vi "Grid_Main_dev.vi"(9 "DC images in":dbl[][][](array[numeric]), 10 "Part of multigrid":bool, 11 "Settings":T3={"Drift Correction Settings"={"Drift Correction every"=80, "Drift correction Pixels"=256, "Channel index (0-23)"=0, "MaxImagesBack"=2, "Threshold"=2, "Increment"=8, "max applied Drift Correction"=20, "Correct Drift"=TRUE, "Correlate"=0, "Correct z drift"=FALSE, "zdrift \nDuration (s)"=0.0}, "Spectroscopy Setting"={"Imaging Current"=1e-11, "ref Current"=7e-11, "tip Speed (m/s)"=2e-09, "Imaging Bias"=0.02, "ref Bias"=-0.1, "preSTS delay [ms]"=500, "STS z offset"=2e-10, "during Spec Bias (V)"=-0.1, "trigger1 < Hz"=0.0, "trigger 2 >Hz"=0.0, "autoStop"=FALSE, "Spectroscopy"=0, "PLL ON/OFF"=TRUE, "readjust setpoint every "=1, "z Reference (constHeight)"=FALSE, "Lock In"=TRUE}, "Misc"={"File name"="symmetric_node_zOff=200p", "Email when finished"="cornelius.krull@monash.edu,Dhaneesh.Gopalakrishnan@monash.edu,marina.castelli@monash.edu"}, "Grid Settings"={"type"=1, "type order"=1, "X pixel"=0, "Y pixel"=0, "Grid_Parms"={"center X (m)"=0.0, "center Y (m)"=0.0, "width (m)"=0.0, "height (m)"=0.0, "angle (deg)"=0.0}}} {"Grid Settings"."type order" items=["Grid", "Random", "Adam7"]; "Grid Settings"."type" items=["Line", "Grid", "Cloud"]; "Spectroscopy Setting"."Spectroscopy" items=["Bias", "zSpec"]; "Spectroscopy Setting"."trigger 2 >Hz" format="%#_6p"; "Spectroscopy Setting"."trigger1 < Hz" format="%#_6p"; "Spectroscopy Setting"."during Spec Bias (V)" format="%#_5p"; "Spectroscopy Setting"."STS z offset" format="%#_6p"; "Spectroscopy Setting"."ref Bias" format="%#_6p"; "Spectroscopy Setting"."Imaging Bias" format="%#_6p"; "Spectroscopy Setting"."tip Speed (m/s)" format="%.2p"; "Spectroscopy Setting"."ref Current" format="%#_6p"; "Spectroscopy Setting"."Imaging Current" format="%#_6p"; "Drift Correction Settings"."Correlate" items=["first Frame", "successive Frames"]; "Drift Correction Settings"."max applied Drift Correction" min=1 max=100 step=1 format="%.0p"; "Drift Correction Settings"."Threshold" min=1 step=1; "Drift Correction Settings"."Channel index (0-23)" items=["Current"=0, "Z (m)"=14]}) -> (1 "DC images out":dbl[][][](array[numeric]), 3 "Settings out":T2)   [LabVIEW 2014]
uses:
  <userlib>/Nanonis Prog Interface V5/Nanonis Prog Interface.lvlib
panel:
  in  "topo_pixel":i32
  in  "resume":T1
  in  "stop":bool
  out "total points":i32
  out "Points taken":i32
  out "ETA":timestamp=timestamp(3575267058.899443 s since 1904-01-01)
  out "remaining time":dbl format="%<%H:%M:%S>t"
  out "Progress":u8(slide)=100 scale=0.0..100.0 scale format="%#.1g"
  out "Last z adjustment":dbl
  out "Last Drift detected (images back)":i32
  out "Y Offset out":sgl format="%#_6p"
  out "X Offset out":sgl format="%#_6p"
  out "Drift Correction Image":picture
  # "RUN smart tilt before starting the GRID\nCHECK CUTOFF\nmove tip to reference point for tip height"
  # "%"
  # "finish the last action and then"
  # "GRID points"
  # "Increase this if no Drift was detected for \na certain number of images"
  # "% of image size"
  # "Only first frame works"
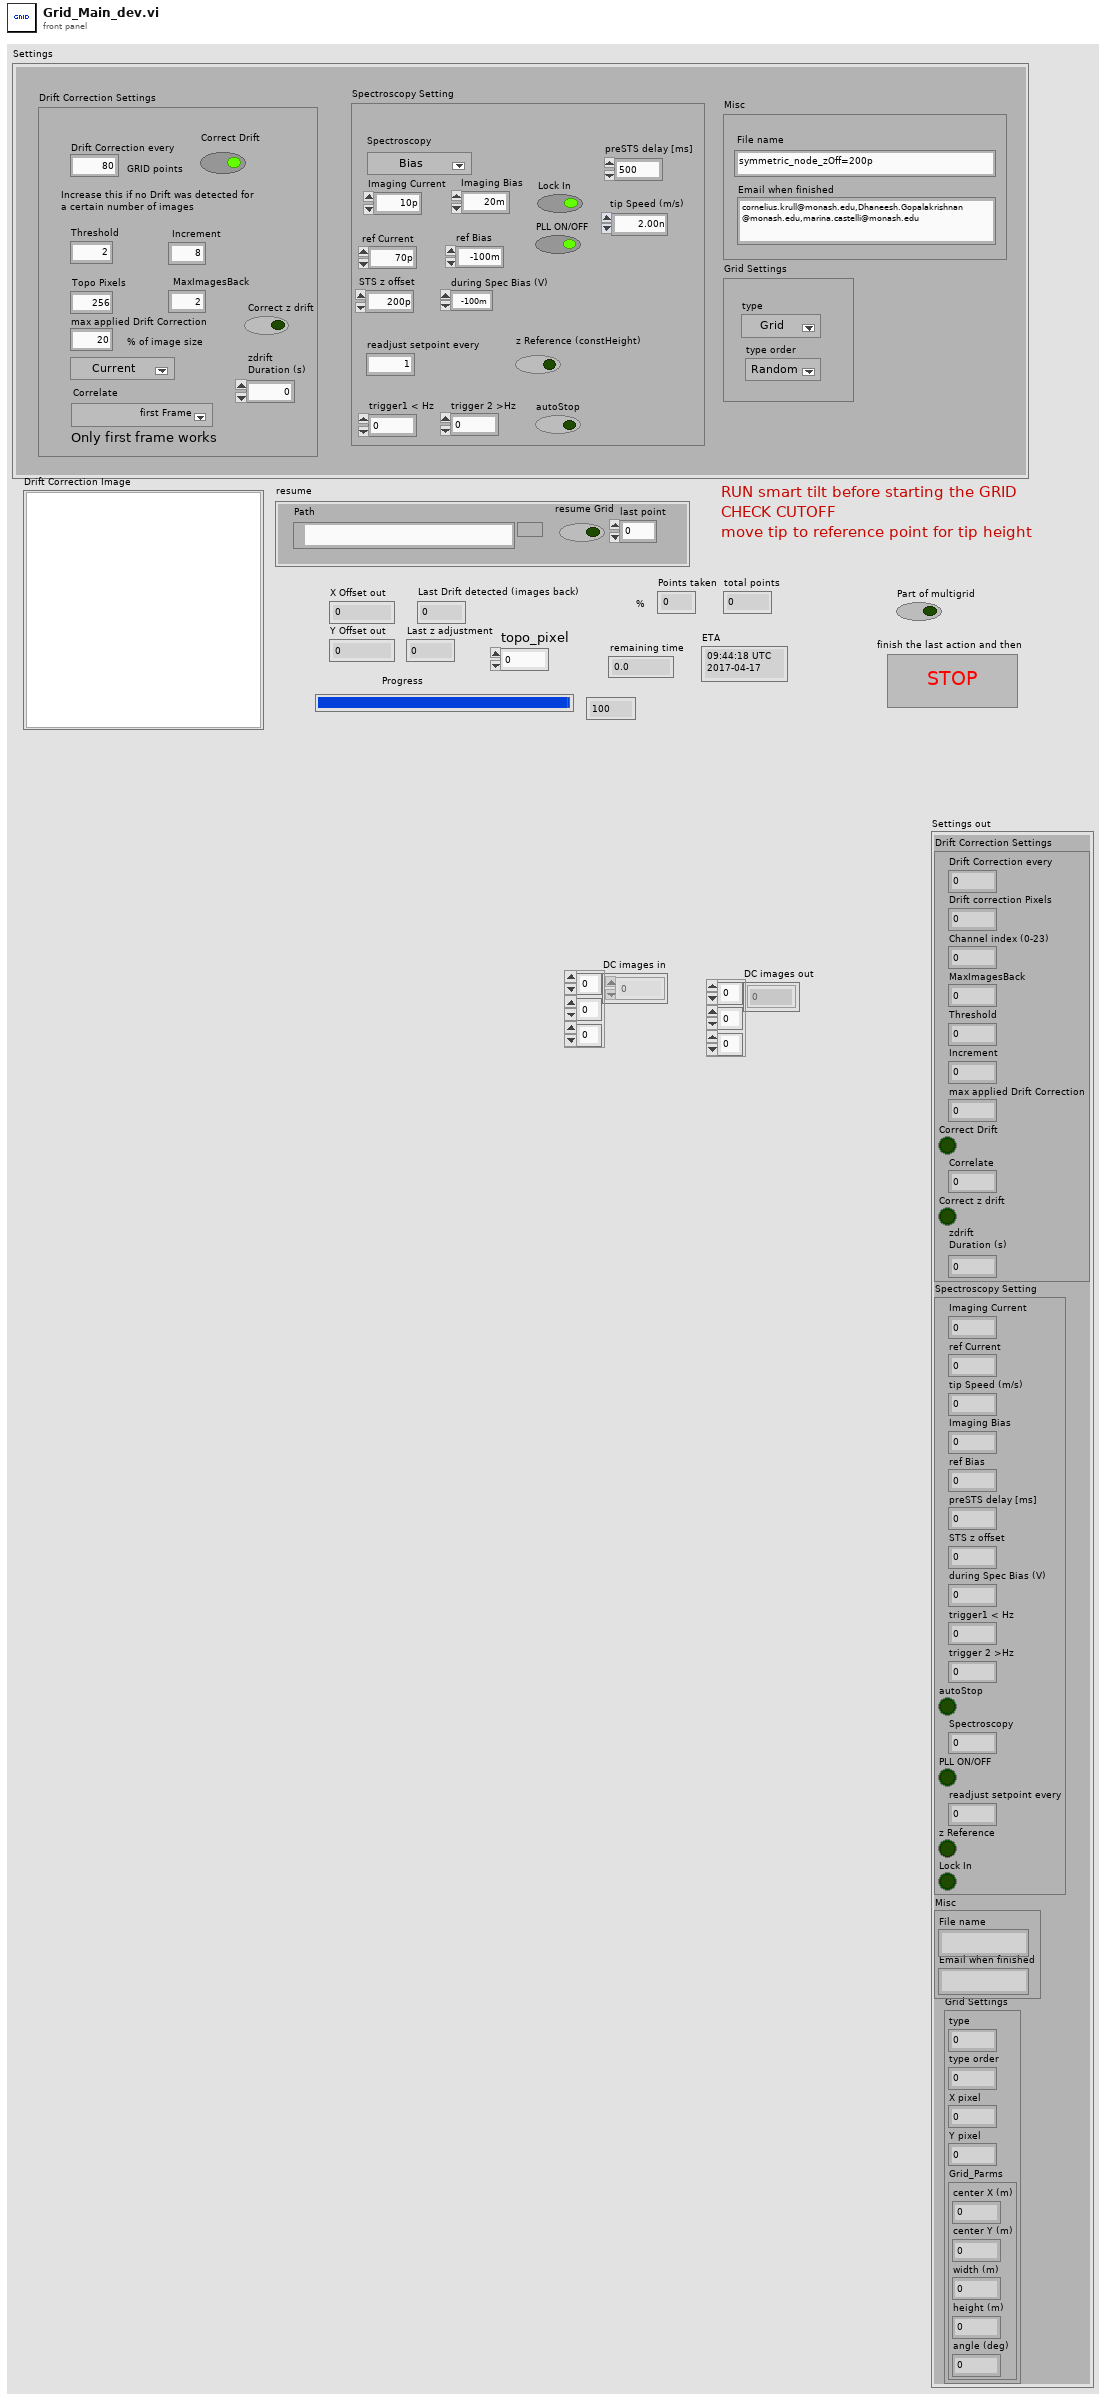
[diagram p1: front panel]
types:
  T1 = cluster{"resume Grid":bool, "Path":path, "last point":i32}
  T2 = cluster{"Drift Correction Settings":cluster{"Drift Correction every":i32, "Drift correction Pixels":i32, "Channel index (0-23)":u8, "MaxImagesBack":i32, "Threshold":i32, "Increment":i32, "max applied Drift Correction":i32, "Correct Drift":bool, "Correlate":u16, "Correct z drift":bool, "zdrift \nDuration (s)":dbl}, "Spectroscopy Setting":cluster{"Imaging Current":dbl, "ref Current":dbl, "tip Speed (m/s)":sgl, "Imaging Bias":dbl, "ref Bias":dbl, "preSTS delay [ms]":u32, "STS z offset":dbl, "during Spec Bias (V)":sgl, "trigger1 < Hz":sgl, "trigger 2 >Hz":sgl, "autoStop":bool, "Spectroscopy":u16, "PLL ON/OFF":bool, "readjust setpoint every ":i32, "z Reference":bool, "Lock In":bool}, "Misc":cluster{"File name":string, "Email when finished":string}, "Grid Settings":cluster{"type":u16, "type order":u16, "X pixel":i32, "Y pixel":i32, "Grid_Parms":cluster{"center X (m)":sgl, "center Y (m)":sgl, "width (m)":sgl, "height (m)":sgl, "angle (deg)":sgl}}}
  T3 = cluster{"Drift Correction Settings":cluster{"Drift Correction every":i32, "Drift correction Pixels":i32, "Channel index (0-23)":u8, "MaxImagesBack":i32, "Threshold":i32, "Increment":i32, "max applied Drift Correction":i32, "Correct Drift":bool, "Correlate":u16, "Correct z drift":bool, "zdrift \nDuration (s)":dbl}, "Spectroscopy Setting":cluster{"Imaging Current":dbl, "ref Current":dbl, "tip Speed (m/s)":sgl, "Imaging Bias":dbl, "ref Bias":dbl, "preSTS delay [ms]":u32, "STS z offset":dbl, "during Spec Bias (V)":sgl, "trigger1 < Hz":sgl, "trigger 2 >Hz":sgl, "autoStop":bool, "Spectroscopy":u16, "PLL ON/OFF":bool, "readjust setpoint every ":i32, "z Reference (constHeight)":bool, "Lock In":bool}, "Misc":cluster{"File name":string, "Email when finished":string}, "Grid Settings":cluster{"type":u16, "type order":u16, "X pixel":i32, "Y pixel":i32, "Grid_Parms":cluster{"center X (m)":sgl, "center Y (m)":sgl, "width (m)":sgl, "height (m)":sgl, "angle (deg)":sgl}}}
  T4 = cluster{"Drift File out":refnum<file>, "zFile":refnum<file>, "BinFile ref":refnum<file>, "xyFile":refnum<file>}
  T5 = cluster{"Drift Correction every":i32, "Drift correction Pixels":i32, "Channel index (0-23)":u8, "MaxImagesBack":i32, "Threshold":i32, "Increment":i32, "max applied Drift Correction":i32, "Correct Drift":bool, "Correlate":u16, "Correct z drift":bool, "zdrift \nDuration (s)":dbl}
  T6 = cluster{"Imaging Current":dbl, "ref Current":dbl, "tip Speed (m/s)":sgl, "Imaging Bias":dbl, "ref Bias":dbl, "preSTS delay [ms]":u32, "STS z offset":dbl, "during Spec Bias (V)":sgl, "trigger1 < Hz":sgl, "trigger 2 >Hz":sgl, "autoStop":bool, "Spectroscopy":u16, "PLL ON/OFF":bool, "readjust setpoint every ":i32, "z Reference":bool, "Lock In":bool}
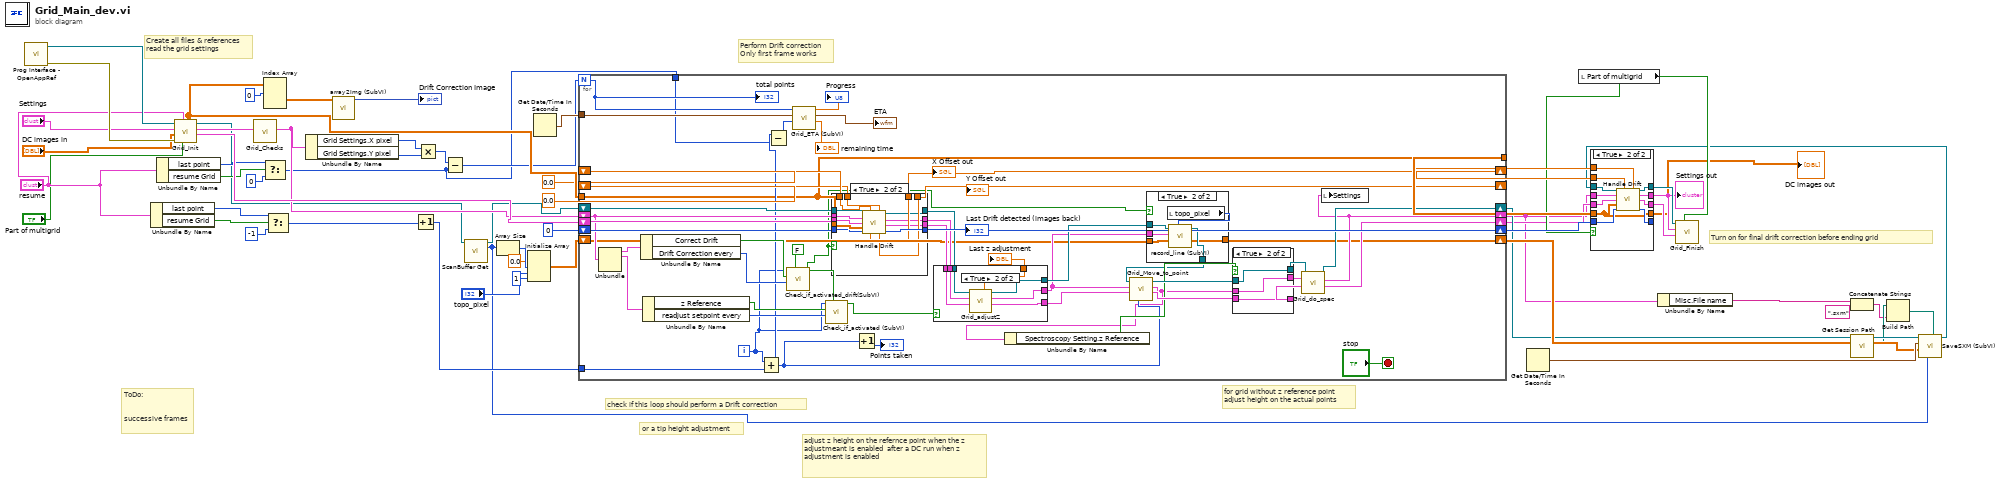
[diagram p0: block diagram]
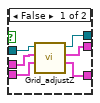
[diagram p4: hidden frame]
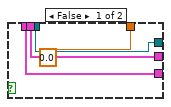
[diagram p5: hidden frame]
diagram:
  # "Turn on for final drift correction before ending grid"
  # "ToDo:\n\n\nsuccessive frames"
  # "Perform Drift correction\nOnly first frame works"
  # "check if this loop should perform a Drift correction"
  # "for grid without z reference point \nadjust height on the actual points"
  # "or a tip height adjustment"
  # "Create all files & references\nread the grid settings"
  # "adjust z height on the refernce point when the z adjustmeant is enabled  after a DC run when z adjustment is enabled"
  n1 = call <userlib>:"Prog Interface - OpenAppRef.vi"() -> ("Error out"=w58:errorcluster, "Application reference"=w59:refnum<vi>)  [unwired: 6 in]
  n2 = Unbundle By Name("resume") -> ("last point"=w41:i32, "resume Grid"=w43:bool)
  n3 = Unbundle By Name("resume") -> ("last point"=w35:i32, "resume Grid"=w37:bool)
  n4 = call "Grid_Init.vi"("Part of multigrid"="Part of multigrid", "resume"="resume", "Error in"=w58, "DC images in"="DC images in", "Settings"="Settings", "Application reference"=w59) -> ("FileRefs"=w56:T4, "Settings out"=w46:T2, "Application ref out"=w18:refnum<vi>, "DC images out"=w54:dbl[][][])  [unwired: 1 in, 1 out]
  n5 = call "Grid_Checks.vi"("Settings"=w46) -> ("Settings out"=w45:T2)  [unwired: 10 in]
  n6 = Index Array(array=w54, index (dim 0)=0 ("index (page)")) -> (element=w55:dbl[][])  [unwired: 2 in]
  n7 = Select(t=w35, s=w37, f=0) -> (s? t:f=w32:i32)
  n8 = Select(t=w41, s=w43, f=-1) -> (s? t:f=w40:i32)
  n9 = Unbundle By Name(w45) -> ("Grid Settings.X pixel"=w49:i32, "Grid Settings.Y pixel"=w48:i32)
  n10 = call "array2Img (SubVI).vi"("Rxy"=w55) -> ("new picture"=→"Drift Correction Image":picture)  [unwired: 10 in]
  n11 = Increment(x=w40) -> (x+1=w38:i32)
  n12 = Multiply(x=w49, y=w48) -> (x*y=w33:i32)
  n13 = Subtract(x=w33, y=w32) -> (x-y=w39:i32)
  n14 = call <userlib>:"ScanBuffer Get.vi"("Application ref in"=w18) -> ("Application ref out"=w17:refnum<vi>, "Channels indexes (0-23)"=w11:i32[])  [unwired: 10 in, 3 out]
  n15 = Array Size(array=w11) -> (size(s)=w20:i32)
  n16 = Initialize Array(0.0 ("element"), w20, "topo_pixel", 1 ("dimension size")) -> (w14:dbl[][][])
  n17 = Get Date/Time In Seconds() -> (seconds since 1Jan1904=w47:timestamp)
  n18 = for {
    N: w39 -> [w73]
    tunnel: w54 -> [w67]
    shift-right: [w108] -> w30
    shift-left: 0 ("Last Drift out") -> [w107]
    shift-right: [w103] -> w28
    shift-left: sgl 0.0 ("X Offset out") -> [w106]
    shift-right: [w104] -> w27
    shift-left: sgl 0.0 ("Y Offset out") -> [w105]
    tunnel: w47 -> [w95]
    shift-right: [w93] -> w9
    shift-left: w17 -> [w109]
    shift-right: [w69] -> w4
    shift-left: w45 -> [w80]
    shift-right: [w92] -> w5
    shift-left: w56 -> [w110]
    tunnel: w38 -> [w81]
    tunnel: w32 -> [w70]
    tunnel: [w67] -> w29
    shift-right: [w62] -> w12
    shift-left: w14 -> [w61]
    i -> [w66]
    stop <- "stop" stop-if-true
    n19 = Unbundle(w80) -> ("Drift Correction Settings"=w79:T5, "Spectroscopy Setting"=w77:T6)  [unwired: 2 out]
    n20 = Unbundle By Name(w79) -> ("Correct Drift"=w78:bool, "Drift Correction every"=w74:i32)
    n21 = Unbundle By Name(w77) -> ("z Reference"=w76:bool, "readjust setpoint every"=w75:i32)
    n22 = Add(x=w66, y=w81) -> (x+y=w71:i32)
    n23 = Subtract(x=w71, y=w70) -> (x-y=w72:i32)
    n24 = call "Check_if_activated_drift(SubVI).vi"("Override"=FALSE, "activate  every  iterations"=w74, "activated?"=w78, "Iteration"=w66) -> ("perform action"=w60:bool)  [unwired: 7 in]
    n25 = call "Grid_ETA (SubVI).vi"("points taken"=w72, "seconds since 1Jan1904"=w95, "points todo"=w73) -> ("Numeric 4"=→"remaining time":dbl, "Time Stamp"=→"ETA":timestamp, "Numeric 3"=→"Progress":dbl)  [unwired: 6 in]
    n26 = call "Check_if_activated (SubVI).vi"("Override"=w60, "activate  every  iterations"=w75, "activated?"=w76, "Iteration"=w66) -> ("perform action"=w100:bool)  [unwired: 7 in]
    n27 = case shown="True" w60 {
      tunnel: w80 -> [w141 w157]
      tunnel: w110 -> [w140 w156]
      tunnel: w109 -> [w139 w155]
      tunnel: w67 -> [_ w154]
      tunnel: [w142 w153] -> w108
      tunnel: w107 -> [w142 w152]
      tunnel: w106 -> [w144 w151]
      tunnel: w105 -> [w143 w150]
      tunnel: [w143 w149] -> w104
      tunnel: [w144 w148] -> w103
      tunnel: [w139 w145] -> w102
      tunnel: [w141 w147] -> w83
      tunnel: [w140 w146] -> w101
      frame False {
      }
      frame True {
        n28 = call "Handle Drift.vi"("Application ref in"=w155, "X Offset in"=w151, "Y Offset In"=w150, "Settings"=w157, "FileRefs"=w156, "Drift Correction image"=w154, "Last Drift"=w152) -> ("Application out"=w145:refnum<vi>, "Settings out"=w147:T2, "FileRefs out File Refs  Out"=w146:T4, "X Offset out"=w148:sgl, "Y Offset out"=w149:sgl, "Last Drift out"=w153:i32)  [unwired: 3 in]
      }
    }
    "X Offset out" <- w103
    "Y Offset out" <- w104
    "Last Drift detected (images back)" <- w108
    n29 = Increment(x=w71) -> (x+1=→"Points taken":i32)
    n30 = case shown="True" w100 {
      tunnel: w102 -> [w130 w138]
      tunnel: w101 -> [w129 w137]
      tunnel: w83 -> [w128 w132]
      tunnel: [w129 w136] -> w94
      tunnel: [w128 w135] -> w63
      tunnel: [w130 w134] -> w65
      tunnel: [0.0 ("Last z adjustment") w133] -> w91
      frame False {
      }
      frame True {
        n31 = call "Grid_adjustZ.vi"("FileRefs"=w137, "Settings"=w132, "Application in"=w138) -> ("FileRefs out"=w136:T4, "Settings out"=w135:T2, "Application ref out"=w134:refnum<vi>, "Last z adjustment"=w133:dbl)  [unwired: 4 in, 1 out]
      }
    }
    "Last z adjustment" <- w91
    n32 = case shown="True" w60 {
      tunnel: w65 -> [w112 w116]
      tunnel: [w112 w118] -> w64
      tunnel: w63 -> [_ w117]
      tunnel: [w111 w115] -> w62
      tunnel: w61 -> [w111 w114]
      frame False {
      }
      frame True {
        n33 = local read "topo_pixel"() -> (w113:i32)
        n34 = call "record_line (SubVI).vi"("topo_pixel"=w113, "Data_in"=w114, "Settings in"=w117, "Application in"=w116) -> ("Data_out"=w115:sgl[][][], "Application out"=w118:refnum<vi>)  [unwired: 5 in, 1 out]
      }
    }
    n35 = call "Grid_Move_to_point.vi"("point"=w71, "FileRefs in"=w94, "Settings"=w63, "Application ref in"=w64) -> ("FileRefs out"=w86:T4, "Settings out"=w68:T2, "Application ref out"=w87:refnum<vi>)  [unwired: 5 in]
    n36 = Unbundle By Name(w68) -> ("Spectroscopy Setting.z Reference"=w85:bool)
    n37 = case shown="True" w85 {
      tunnel: [w124 w127] -> w90
      tunnel: [w123 w125] -> w88
      tunnel: [w122 w126] -> w89
      tunnel: w87 -> [w121 w127]
      tunnel: w68 -> [w120 w126]
      tunnel: w86 -> [w119 w125]
      frame False {
        n38 = call "Grid_adjustZ.vi"("FileRefs"=w119, "Settings"=w120, "Application in"=w121) -> ("FileRefs out"=w123:T4, "Settings out"=w122:T2, "Application ref out"=w124:refnum<vi>)  [unwired: 4 in, 2 out]
      }
      frame True {
      }
    }
    n39 = call "Grid_do_spec.vi"("FileRefs in"=w88, "Settings in"=w89, "Application ref in"=w90) -> ("FileRefs out"=w92:T4, "Settings out"=w69:T2, "Application ref out"=w93:refnum<vi>)  [unwired: 5 in, 1 out]
    n40 = local write "Settings"(w69) -> ()
    "total points" <- w73
  }
  n41 = Get Date/Time In Seconds() -> (seconds since 1Jan1904=w13:timestamp)
  n42 = local read "Part of multigrid"() -> (w24:bool)
  n43 = Unbundle By Name(w4) -> ("Misc.File name"=w3:string)
  n44 = Concatenate Strings(w3, ".sxm" ("string")) -> (w2:string)
  n45 = call <userlib>:"Get Session Path.vi"("Application ref in"=w9) -> ("Session path"=w7:path, "Application ref out"=w8:refnum<vi>)  [unwired: 8 in, 1 out]
  n46 = Build Path(base path=w7, name or relative path=w2) -> (appended path=w6:path)
  n47 = call "SaveSXM (SubVI).vi"("Application ref in"=w8, "seconds since 1Jan1904"=w13, "DataIn"=w12, "Channels indexes (0-23)"=w11, "selected path"=w6) -> ("Application ref out"=w10:refnum<vi>)  [unwired: 4 in, 1 out]
  n48 = case shown="True" w24 {
    tunnel: w4 -> [w161 w173]
    tunnel: w5 -> [w160 w172]
    tunnel: w10 -> [w159 w171]
    tunnel: [w162 w170] -> _
    tunnel: w30 -> [w162 w166]
    tunnel: [w159 w169] -> w31
    tunnel: [w161 w168] -> w25
    tunnel: [w160 w167] -> w26
    tunnel: w29 -> [w158 w163]
    tunnel: w28 -> [_ w165]
    tunnel: w27 -> [_ w164]
    tunnel: [w158 w163] -> w22
    frame False {
    }
    frame True {
      n49 = call "Handle Drift.vi"("Application ref in"=w171, "X Offset in"=w165, "Y Offset In"=w164, "Settings"=w173, "FileRefs"=w172, "Drift Correction image"=w163, "Last Drift"=w166) -> ("Application out"=w169:refnum<vi>, "Settings out"=w168:T2, "FileRefs out File Refs  Out"=w167:T4, "Last Drift out"=w170:i32)  [unwired: 3 in, 2 out]
    }
  }
  "Settings out" <- w25
  "DC images out" <- w22
  n50 = call "Grid_Finish.vi"("Part of multigrid"=w24, "FileRefs"=w26, "Settings"=w25, "Application reference"=w31) -> ()  [unwired: 8 in]
